vi "MT Bit Stream to Digital Graph.vi"(6 "Reset (F)":bool, 7 "Format":enum16{"single plot", "plot per bit"}(ring), 9 "Symbol Rate (Hz)":dbl=1.0 format="%.2f", 10 "bits per symbol":i32=1, 11 "Bit Stream":i8[](array[numeric])) -> (3 "Digital Waveform Graph":T1(graph))   [LabVIEW 2020, in "niDMT.lvlib"]
uses:
  <vilib>/addons/Modulation/niDMT.lvlib
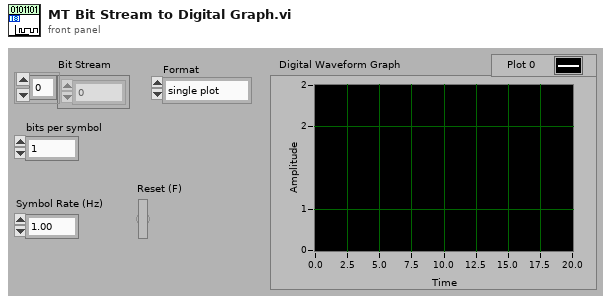
[diagram p1: front panel]
types:
  T1 = cluster{cluster{"1/x":dbl, dbl, i8[], i32}, i32[][]}
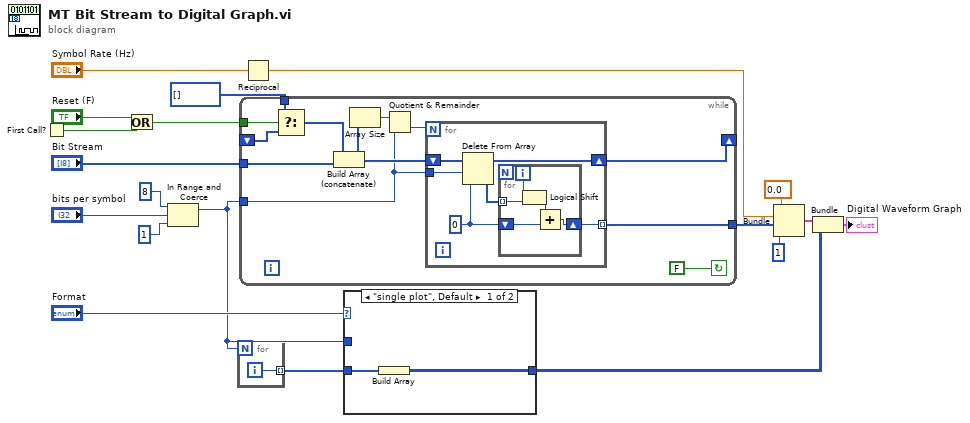
[diagram p0: block diagram]
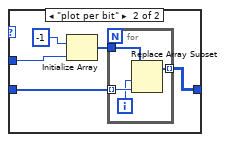
[diagram p2: hidden frame]
diagram:
  n1 = First Call?() -> (First Call?: T/F=w4:bool)
  n2 = Or(x="Reset (F)", y=w4) -> (x .or. y?=w3:bool)
  n3 = In Range and Coerce(upper limit=8, x="bits per symbol", lower limit=1) -> (coerced(x)=w1:i32)  [unwired: 1 out]
  n4 = for {
    N: w1 -> [_]
    tunnel: [w20] -> w9 mode=indexing
    i -> [w20]
  }
  n5 = while {
    tunnel: w1 -> [w27]
    tunnel: "Bit Stream" -> [w31]
    shift-right: [w30] -> _
    shift-left: _ -> [w22]
    tunnel: [w26] -> w17
    tunnel: w3 -> [w24]
    tunnel: i8[] [] -> [w23]
    stop <- FALSE continue-if-true
    n6 = Select(t=w23, s=w24, f=w22) -> (s? t:f=w21:i8[])
    n7 = Build Array (concatenate)(w21, w31) -> (w28:i8[])
    n8 = Array Size(array=w28) -> (size(s)=w29:i32)
    n9 = Quotient & Remainder(x=w29, y=w27) -> (floor(x/y)=w32:i32)  [unwired: 1 out]
    n10 = for {
      N: w32 -> [_]
      shift-right: [w36] -> w30
      shift-left: w28 -> [w38]
      tunnel: w27 -> [w37]
      tunnel: [w34] -> w26 mode=indexing
      w33 = i8 0
      n11 = Delete From Array(array=w38, length=w37, index=w33) -> (deleted portion=w35:i8[], array with subset deleted=w36:i8[])
      n12 = for {
        tunnel: w35 -> [w43] mode=indexing
        shift-right: [w41] -> w34
        shift-left: w33 -> [w39]
        i -> [w42]
        n13 = Logical Shift(y=w42, x=w43) -> (x << y=w40:i8)
        n14 = Add(x=w40, y=w39) -> (x+y=w41:i8)
      }
    }
  }
  n15 = Reciprocal(x="Symbol Rate (Hz)") -> (1/x=w16:dbl)
  n16 = case shown="\"single plot\", Default" "Format" {
    tunnel: [w44 w47] -> w11
    tunnel: w9 -> [w45 w48]
    tunnel: w1 -> [_ w46]
    frame "single plot", Default {
      n17 = Build Array(w45) -> (w44:i32[][])
    }
    frame "plot per bit" {
      n18 = Initialize Array(-1 ("element"), w46) -> (w49:i32[])
      n19 = for {
        tunnel: w49 -> [w52]
        tunnel: w48 -> [w54] mode=indexing
        tunnel: [w51] -> w47 mode=indexing
        i -> [w53]
        n20 = Replace Array Subset(array=w52, new element=w54, index=w53) -> (w51:i32[])
      }
    }
  }
  n21 = Bundle("1/x"=0.0, w16, w17, 1) -> (w12:cluster{"1/x":dbl, dbl, i8[], i32})  [unwired: 1 out]
  n22 = Bundle(w12, w11) -> (→"Digital Waveform Graph":T1)  [unwired: 1 out]
